vi "UpdateFPReply.vi"(1 "success?":bool, 2 "Reply":string, 3 "Sent":string, 4 "method":string) -> (0 "Log":T1)   [LabVIEW 2010]
uses:
  _ROSDefinition.vi
  Servers/ServerSubs/ROSLog.ctl
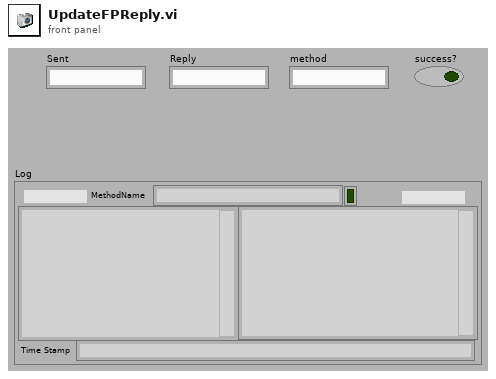
[diagram p1: front panel]
types:
  T1 = typedef "ROSLog.ctl" = cluster{"Sent":string, "Reply":string, "MethodName":string, "success":bool, "Dir1":string, "Dir2":string, "Time Stamp":string}
  T2 = cluster{"Sent":string, "Reply":string, "method":string, "success?":bool, "element":string, "element":string, "Current Time":string}
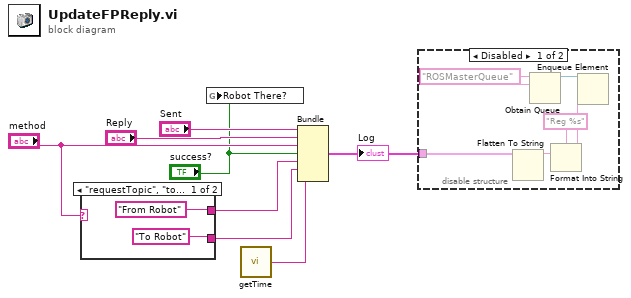
[diagram p0: block diagram]
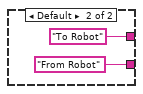
[diagram p2: hidden frame]
diagram:
  n1 = case shown="\"requestTopic\", \"topicReply\"" "method" {
    tunnel: ["From Robot" ("element") "To Robot" ("element")] -> w5
    tunnel: ["To Robot" ("element") "From Robot" ("element")] -> w4
    frame "requestTopic", "topicReply" {
    }
    frame Default {
    }
  }
  n2 = global write "_ROSDefinition.vi" "Robot There?"("success?") -> ()
  n3 = call "getTime.vi"() -> ("Current Time"=w3:string)  [unwired: 1 in]
  n4 = Bundle("Sent"="Sent", "Reply"="Reply", "method"="method", "success?"="success?", "element"=w5, "element"=w4, "Current Time"=w3) -> (w8:T2)  [unwired: 1 in]
  "Log" <- w8
  n5 = disable-structure shown="Disabled" {
    disable-tunnel: w8 -> [w16 _]
    frame Disabled {
      w13 = "ROSMasterQueue" ("name (unnamed)")
      n6 = Flatten To String(anything=w16) -> (data string=w17:string)  [unwired: 3 in, 2 out]
      n7 = Obtain Queue(name (unnamed)=w13, element data type=w13) -> (queue out=w14:refnum<queue>)  [unwired: 3 in, 2 out]
      n8 = Format Into String(format string="Reg %s" ("element"), w17) -> (resulting string=w18:string)  [unwired: 2 in, 1 out]
      n9 = Enqueue Element(queue=w14, element=w18) -> ()  [unwired: 2 in, 3 out]
    }
    frame Enabled {
    }
  }
